vi "Read Register.vi"(6 "Read Delay ms (5)":u32=5, 7 "SPI Connection":refnum<class "SPI Connection.lvclass">, 8 "error in (no error)":errorcluster, 9 "Len":u8, 10 "Register":u8 format="%.0x") -> (0 "error out":errorcluster, 1 "Data":string)   [LabVIEW 2024, in "CTI.lvlib" / "SPI Connection.lvclass"]
uses:
  SPI Connection.lvclass
  SPI Connection.lvclass/SPI Connection.ctl
  3f2eec9a-ce11-49d3-a293-9054af33640d.vi
  Session/Session.lvclass
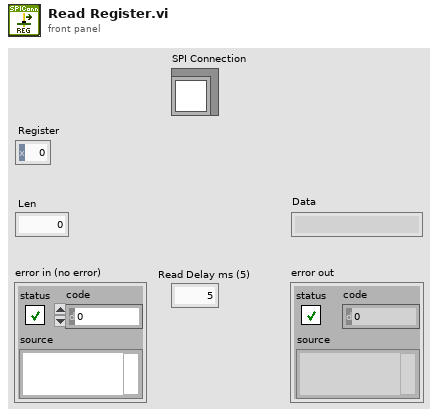
[diagram p1: front panel]
types:
  T1 = typedef "CTI.lvlib/SPI Number.ctl" = i8
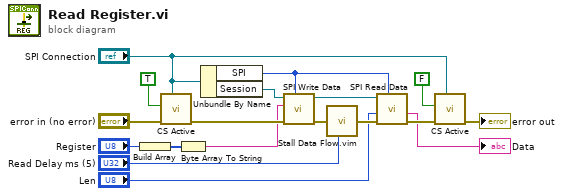
[diagram p0: block diagram]
diagram:
  n1 = Build Array("Register") -> (w15:u8[])
  n2 = call "CS Active.vi"("SPI Connection"="SPI Connection", "error in (no error)"="error in (no error)", "CS Active"=TRUE) -> ("error out"=w17:errorcluster)  [unwired: 8 in]
  n3 = Byte Array To String(unsigned byte array=w15) -> (string=w12:string)
  n4 = Unbundle By Name("SPI Connection") -> ("SPI"=w7:T1, "Session"=w1:refnum<class "Session.lvclass">)
  n5 = call "SPI Write Data.vi"("SPI #"=w7, "error in (no error)"=w17, "Data"=w12, "Session in"=w1) -> ("error out"=w13:errorcluster, "Session out"=w9:refnum<class "Session.lvclass">)  [unwired: 6 in]
  n6 = call "Stall Data Flow.vim"("value in"=w13, "milliseconds to wait"="Read Delay ms (5)") -> ("value out"=w11:errorcluster)  [unwired: 1 out]
  n7 = call "SPI Read Data.vi"("SPI #"=w7, "error in (no error)"=w11, "Len"="Len", "Session in"=w9) -> ("error out"=w5:errorcluster, "Data"=→"Data":string)  [unwired: 5 in, 1 out]
  n8 = call "CS Active.vi"("SPI Connection"="SPI Connection", "error in (no error)"=w5, "CS Active"=FALSE) -> ("error out"=→"error out":errorcluster)  [unwired: 8 in]
